vi "Update Scene Object.vi"(4 "Action":T8, 6 "Control Ref Queue":T1, 7 "Multiplot Representation In":T4, 8 "error in (no error)":errorcluster, 9 "Object Cluster In":T7, 10 "Actual Transform In":T2, 11 "3D Plot.lvclass in":refnum<class "3D Plot.lvclass">) -> (0 "error out":errorcluster, 1 "Object Cluster Out":T7, 2 "Actual Transform Out":T2, 3 "3D Plot.lvclass out":refnum<class "3D Plot.lvclass">, 5 "Multiplot Representation Out":T4)   [LabVIEW 2020, in "3D Plot.lvclass"]
uses:
  <vilib>/Math Plots/3D Math Plots/3D Plot/3D Plot/3D Plot.lvclass
  <vilib>/Math Plots/3D Math Plots/3D Plot/3D Plot/Typedef/Object Cluster.ctl
  <vilib>/Math Plots/3D Math Plots/3D Plot/3D Plot/Typedef/Plot Action.ctl
  <vilib>/Math Plots/3D Math Plots/3D Plot/3D Plot/Typedef/Multiplot Representation.ctl
  <vilib>/Math Plots/3D Math Plots/3D Plot/3D Plot/Typedef/Plot Representation.ctl
  <vilib>/Math Plots/3D Math Plots/3D Plot/3D Plot/Typedef/Range Clusters.ctl
  <vilib>/Math Plots/3D Math Plots/3D Plot/3D Plot/Typedef/Mesh Data.ctl
  <vilib>/Math Plots/3D Math Plots/3D Plot/3D Plot/Typedef/Actual Transform.ctl
  <vilib>/Math Plots/3D Math Plots/3D Plot/Action String/3DMathPlot Ctrl Act Queue.ctl
  <vilib>/Math Plots/3D Math Plots/3D Plot/Action String/3DMathPlot Ctrl Act Cluster.ctl
  <vilib>/Math Plots/3D Math Plots/3D Plot/Action String/3DMathPlot State Class.ctl
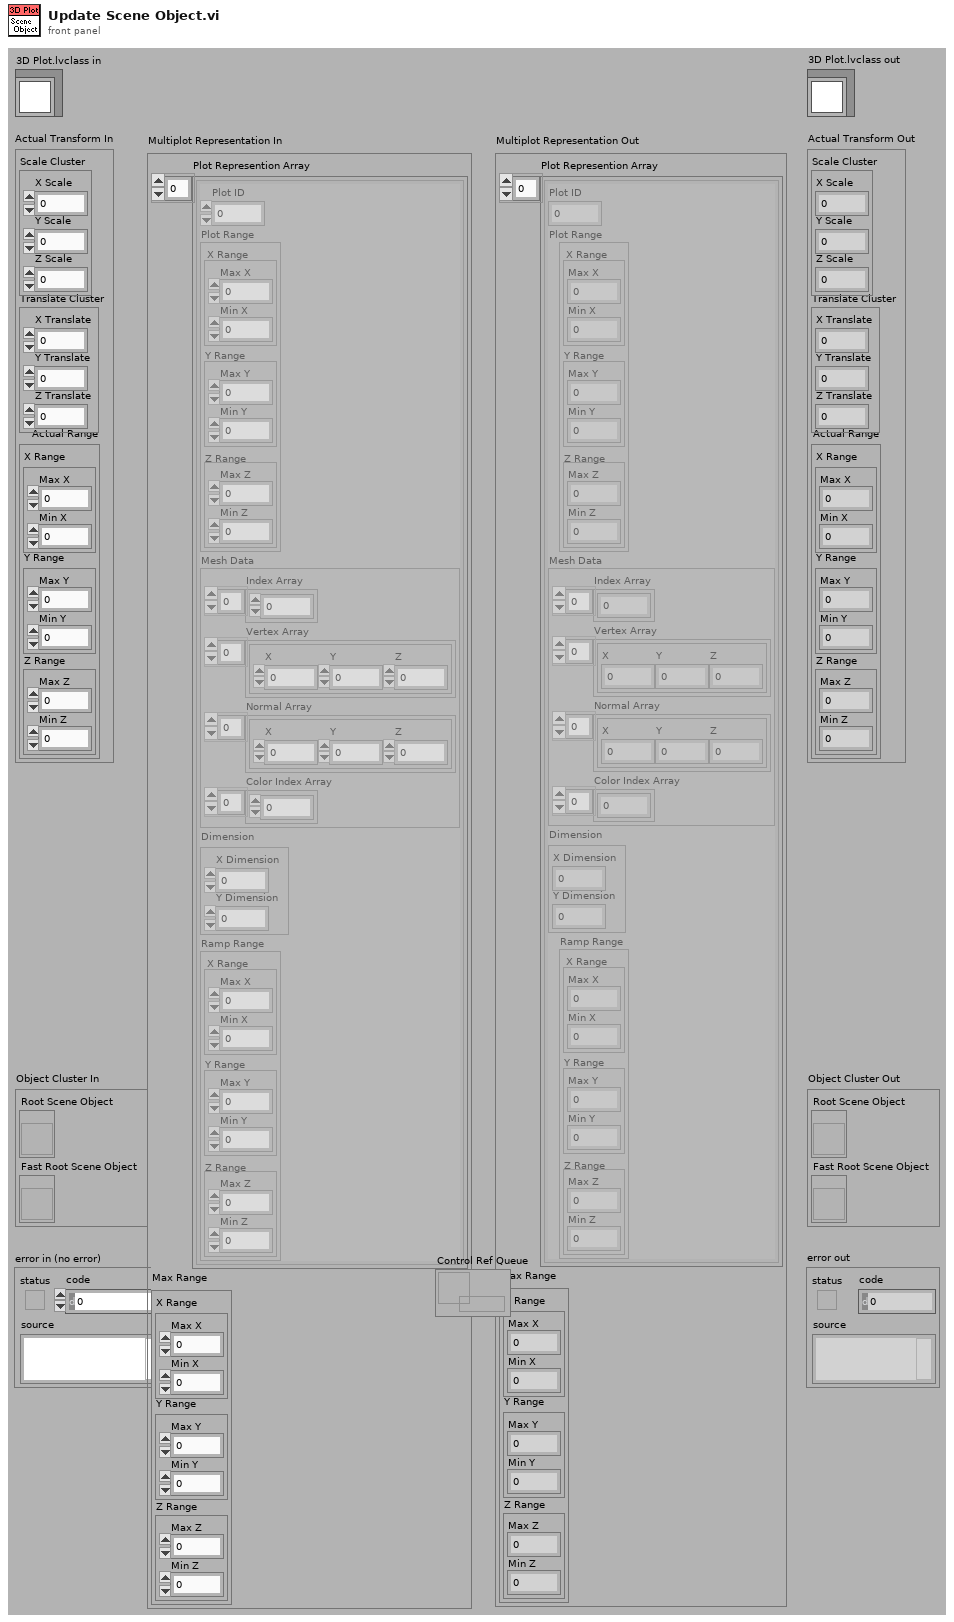
[diagram p1: front panel]
types:
  T1 = typedef "3DMathPlot Ctrl Act Queue.ctl" = refnum<queue>
  T2 = typedef "3D Plot.lvclass/Actual Transform.ctl" = cluster{"Scale Cluster":cluster{"X Scale":sgl, "Y Scale":sgl, "Z Scale":sgl}, "Translate Cluster":cluster{"X Translate":sgl, "Y Translate":sgl, "Z Translate":sgl}, "Actual Range":T3}
  T3 = typedef "3D Plot.lvclass/Range Clusters.ctl" = cluster{"X Range":cluster{"Max X":sgl, "Min X":sgl}, "Y Range":cluster{"Max Y":sgl, "Min Y":sgl}, "Z Range":cluster{"Max Z":sgl, "Min Z":sgl}}
  T4 = typedef "3D Plot.lvclass/Multiplot Representation.ctl" = cluster{"Plot Represention Array":T5[], "Max Range":T3}
  T5 = typedef "3D Plot.lvclass/Plot Representation.ctl" = cluster{"Plot ID":i32, "Plot Range":T3, "Mesh Data":T6, "Dimension":cluster{"X Dimension":i32, "Y Dimension":i32}, "Ramp Range":T3}
  T6 = typedef "3D Plot.lvclass/Mesh Data.ctl" = cluster{"Index Array":u32[], "Vertex Array":cluster{"X":sgl, "Y":sgl, "Z":sgl}[], "Normal Array":cluster{"X":sgl, "Y":sgl, "Z":sgl}[], "Color Index Array":i32[]}
  T7 = typedef "3D Plot.lvclass/Object Cluster.ctl" = cluster{"Root Scene Object":refnum<vi>, "Fast Root Scene Object":refnum<vi>}
  T8 = typedef "3D Plot.lvclass/Plot Action.ctl" = cluster{"Light Action":enum16{"Update", "Remove", "Nothing"}, "Axis Action":enum16{"Update", "Remove", "Nothing"}, "Plot Action":enum16{"Update", "Remove", "Nothing"}, "Cursor Action":enum16{"Update", "Remove", "Nothing"}, "Fast Draw Action":enum16{"Update", "Remove", "Nothing"}}
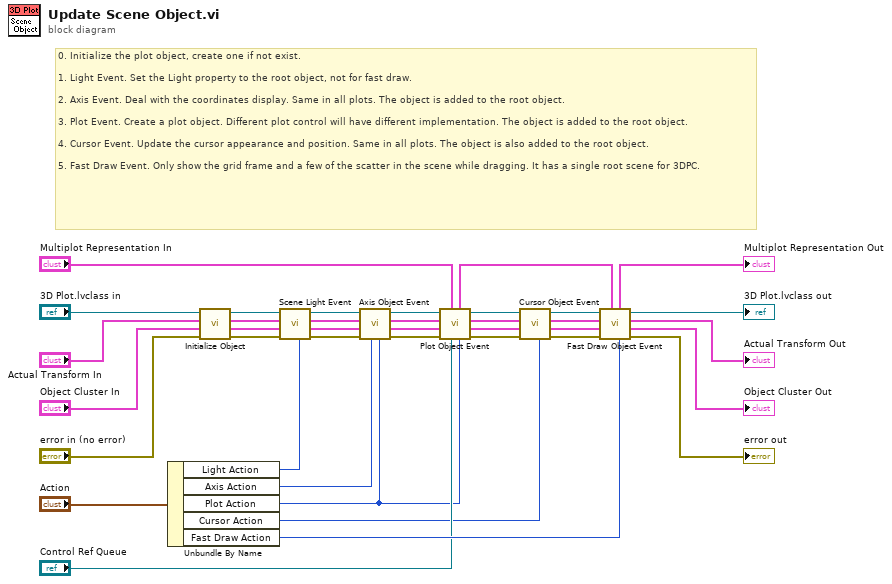
[diagram p0: block diagram]
diagram:
  # "0. Initialize the plot object, create one if not exist. \n\n1. Light Event. Set the Light property to the root object, not for fast draw. \n\n2. Axis Event. Deal with the coordinates display. Same in all plots. The object is added to the root object.\n\n3. Plot Event. Create a plot object. Different plot control will have different implementation. The object is added to the root object.\n\n4. Cursor Event. Update the cursor appearance and position. Same in all plots. The object is also added to the root object.\n\n5. Fast Draw Event. Only show the grid frame and a few of the scatter in the scene while dragging. It has a single root scene for 3DPC."
  n1 = Unbundle By Name("Action") -> ("Light Action"=w28:enum16{"Update", "Remove", "Nothing"}, "Axis Action"=w6:enum16{"Update", "Remove", "Nothing"}, "Plot Action"=w5:enum16{"Update", "Remove", "Nothing"}, "Cursor Action"=w7:enum16{"Update", "Remove", "Nothing"}, "Fast Draw Action"=w27:enum16{"Update", "Remove", "Nothing"})
  n2 = call <vilib>:"Initialize Object.vi"("error in (no error)"="error in (no error)", "Object Cluster In"="Object Cluster In") -> ("error out"=w15:errorcluster, "Object Cluster Out"=w16:T7)  [unwired: 8 out]
  n3 = call <vilib>:"Scene Light Event.vi"("Light Action"=w28, "error in (no error)"=w15, "Object Cluster In"=w16, "3D Plot.lvclass in"="3D Plot.lvclass in") -> ("error out"=w29:errorcluster, "Object Cluster Out"=w30:T7, "3D Plot.lvclass out"=w31:refnum<class "3D Plot.lvclass">)  [unwired: 1 in, 4 out]
  n4 = call <vilib>:"Axis Object Event.vi"("Plot Action"=w5, "Axis Action"=w6, "error in (no error)"=w29, "Object Cluster In"=w30, "Actual Transform In"="Actual Transform In", "3D Plot.lvclass in"=w31) -> ("error out"=w1:errorcluster, "Object Cluster Out"=w2:T7, "Actual Transform Out"=w3:T2, "3D Plot.lvclass out"=w4:refnum<class "3D Plot.lvclass">)  [unwired: 1 in, 1 out]
  n5 = call <vilib>:"Plot Object Event.vi"("Plot Action"=w5, "Control Ref Queue"="Control Ref Queue", "Multiplot Representation In"="Multiplot Representation In", "error in (no error)"=w1, "Object Cluster In"=w2, "Actual Transform In"=w3, "3D Plot.lvclass in"=w4) -> ("error out"=w23:errorcluster, "Object Cluster Out"=w22:T7, "Actual Transform Out"=w13:T2, "3D Plot.lvclass out"=w24:refnum<class "3D Plot.lvclass">, "Multiplot Representation Out"=w9:T4)
  n6 = call <vilib>:"Cursor Object Event.vi"("Cursor Action"=w7, "error in (no error)"=w23, "Object Cluster In"=w22, "Actual Transform In"=w13, "3D Plot.lvclass in"=w24) -> ("error out"=w20:errorcluster, "Object Cluster Out"=w21:T7, "Actual Transform Out"=w12:T2, "3D Plot.lvclass out"=w25:refnum<class "3D Plot.lvclass">)  [unwired: 2 in, 1 out]
  n7 = call <vilib>:"Fast Draw Object Event.vi"("Fast Draw Action"=w27, "Multiplot Representation In"=w9, "error in (no error)"=w20, "Object Cluster In"=w21, "Actual Transform In"=w12, "3D Plot.lvclass in"=w25) -> ("error out"=→"error out":errorcluster, "Object Cluster Out"=→"Object Cluster Out":T7, "Actual Transform Out"=→"Actual Transform Out":T2, "3D Plot.lvclass out"=→"3D Plot.lvclass out":refnum<class "3D Plot.lvclass">, "Multiplot Representation Out"=→"Multiplot Representation Out":T4)  [unwired: 1 in]
